vi "new.vi"(5 "Range in":refnum<class "Block.lvclass">, 8 "error in (no error)":errorcluster, 9 "size":i32) -> (0 "error out":errorcluster, 3 "Range out":refnum<class "Block.lvclass">)   [LabVIEW 2020, in "lvdata.lvlib" / "Block.lvclass"]
uses:
  Block.lvclass
  Block.lvclass/Block.ctl
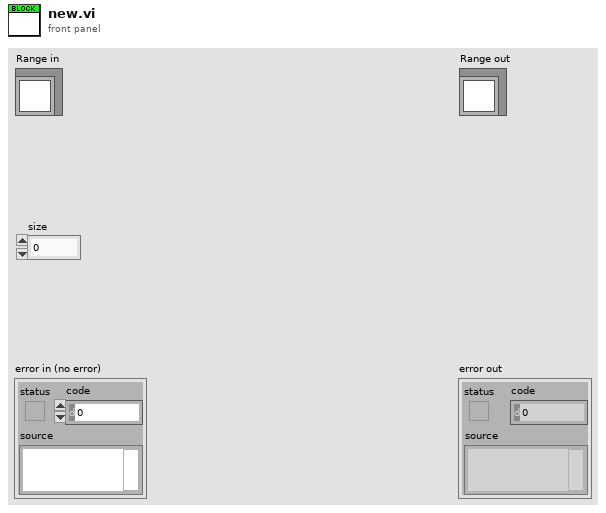
[diagram p1: front panel]
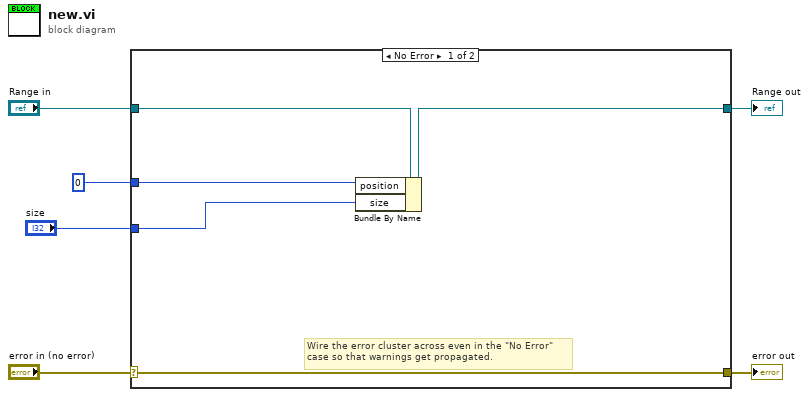
[diagram p0: block diagram]
diagram:
  n1 = case shown="No Error" "error in (no error)" {
    selector: "error in (no error)" -> [w10 w13]
    tunnel: [w10 w13] -> w5
    tunnel: [w9 w12] -> w3
    tunnel: "Range in" -> [w11 w12]
    tunnel: "size" -> [w8 _]
    tunnel: 0 ("position") -> [w7 _]
    frame No Error {
      # "Wire the error cluster across even in the \"No Error\"\ncase so that warnings get propagated."
      n2 = Bundle By Name(cluster=w11, "position"=w7, "size"=w8) -> (w9:refnum<class "Block.lvclass">)
    }
    frame Error {
    }
  }
  "error out" <- w5
  "Range out" <- w3
